vi "Sorting_Array.vi"() -> ()   [LabVIEW 2024]
panel:
  out "Array":dbl[](array[numeric])
  in  "Numeric 5":i32
  out "sorted array":dbl[](array[numeric])
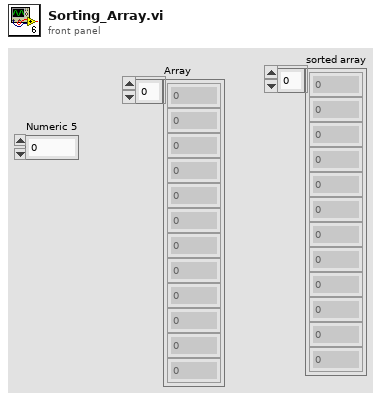
[diagram p1: front panel]
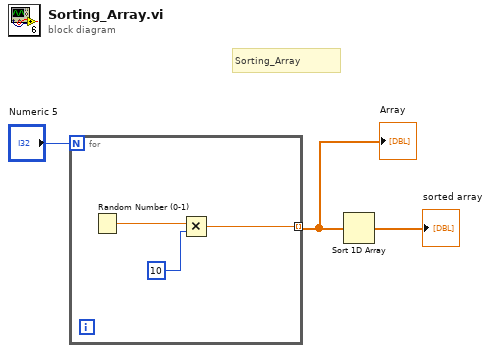
[diagram p0: block diagram]
diagram:
  # "Sorting_Array"
  n1 = for {
    N: "Numeric 5" -> [_]
    tunnel: [w4] -> w1 mode=indexing
    n2 = Random Number (0-1)() -> (number: 0 to 1=w6:dbl)
    n3 = Multiply(x=w6, y=10) -> (x*y=w4:dbl)
  }
  "Array" <- w1
  n4 = Sort 1D Array(array=w1) -> (sorted array=→"sorted array":dbl[])
